vi "Test 3.vi"(8 "error in (no error)":errorcluster, 11 "Test Case In":refnum<class "Tests.lvclass">) -> (0 "error out":errorcluster, 3 "Test Case Out":refnum<class "Tests.lvclass">)   [LabVIEW 2021, in "Tests.lvclass"]
uses:
  Tests.lvclass
  C:/Program Files (x86)/National Instruments/LabVIEW 2021/vi.lib/Astemes/LUnit/Test Case.lvclass
  <vilib>/Astemes/LUnit/Test Case.lvclass/Test Case.ctl
  4993e8ee-a06a-463a-9684-69129f64d5ce.vi
  <vilib>/Astemes/LUnit/Append Pass Result.vi
  <vilib>/Astemes/LUnit/Append Fail Result.vi
  <vilib>/Astemes/LUnit/Compare Variants.vi
  <vilib>/Astemes/LUnit/Describe Comparison of Arrays.vi
  <vilib>/Astemes/LUnit/Variant to string.vi
  <vilib>/AdvancedString/1D String Array to Delimited String.vi
  <vilib>/Utility/Data Type/Get Type Information.vi
  <vilib>/Utility/LVClass/Get LV Class Name.vi
  Proto/Proto.lvclass
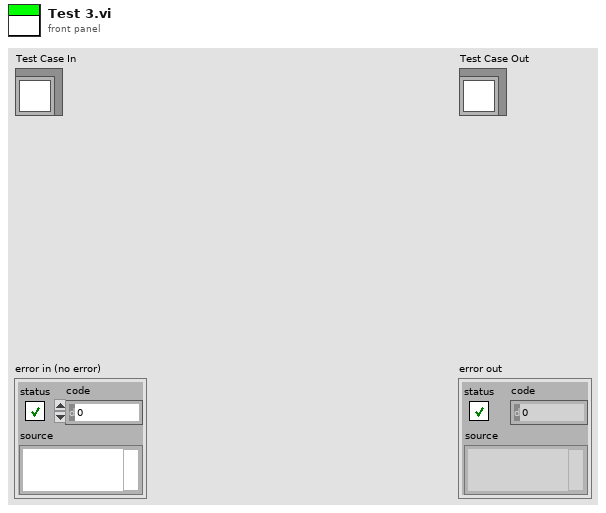
[diagram p1: front panel]
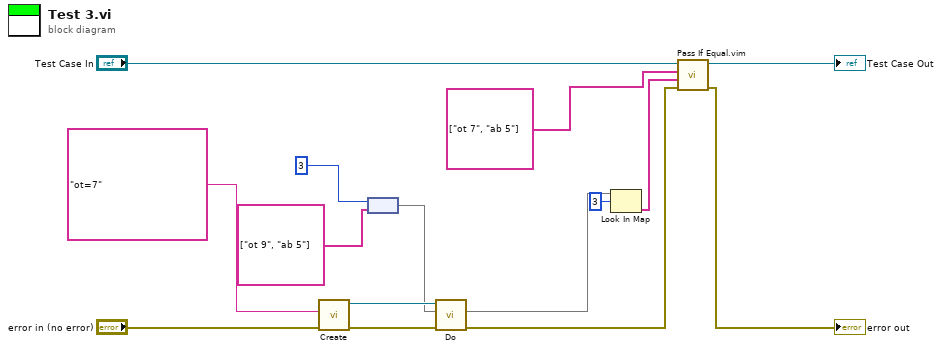
[diagram p0: block diagram]
diagram:
  n1 = call "Create.vi"("error in (no error)"="error in (no error)", "Input"="ot=7") -> ("error out"=w11:errorcluster, "Proto"=w9:refnum<class "Proto.lvclass">)  [unwired: 8 in]
  n2 = node(3 ("dimension size"), string[] ["ot 9", "ab 5"] ("value")) -> (w1:map{i32, string[]})
  n3 = call "Do.vi"("error in (no error)"=w11, "Boxes"=w1, "Proto in"=w9) -> ("error out"=w10:errorcluster, "Boxes out"=w7:map{i32, string[]})  [unwired: 6 in, 1 out]
  n4 = Look In Map(map=w7, key=3) -> (value=w5:string[])  [unwired: 1 in, 1 out]
  n5 = call "Pass If Equal.vim"("error in (no error)"=w10, "Actual"=w5, "Expected"=string[] ["ot 7", "ab 5"] ("value"), "LUnit Test Case In"="Test Case In") -> ("error out"=→"error out":errorcluster, "LUnit Test Case Out"=→"Test Case Out":refnum<class "Tests.lvclass">)  [unwired: 6 in]
